vi "Get Dependencies.vi"(8 "error in (no error)":errorcluster, 11 "Device Ref in":T5 format="%.0x") -> (0 "error out":errorcluster, 2 "Dependencies":T1[](array[typedef]), 3 "Dev Ref out":T5 format="%.0x")   [LabVIEW 2011, in "TDMS Custom Device.lvlib"]
uses:
  TDMS Custom Device.lvlib
  <vilib>/NI Veristand/Custom Device API/Custom Device Item Ref.ctl
  <vilib>/NI Veristand/Custom Device API/Custom Device File Dependency.ctl
  <vilib>/NI Veristand/Custom Device API/Path Specification.ctl
  <vilib>/NI Veristand/Custom Device API/Path Type.ctl
  <vilib>/NI Veristand/Custom Device API/Custom Device Supported Target.ctl
  NationalInstruments.VeriStand.SystemStorage
  <vilib>/NI Veristand/Custom Device API/Custom Device API.lvlib
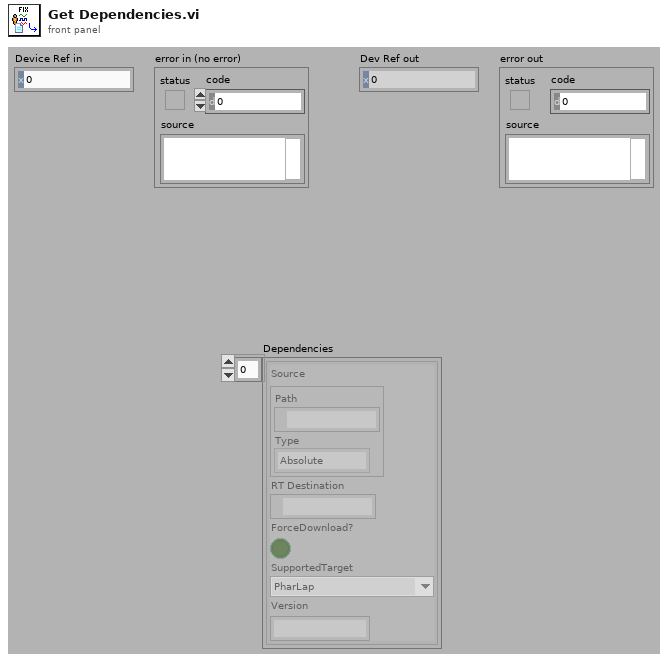
[diagram p1: front panel]
types:
  T1 = typedef "Custom Device API.lvlib/Custom Device File Dependency.ctl" = cluster{"Source":T2, "RT Destination":path, "ForceDownload?":bool, "SupportedTarget":T4, "Version":string}
  T2 = typedef "Custom Device API.lvlib/Path Specification.ctl" = cluster{"Path":path, "Type":T3}
  T3 = typedef "Custom Device API.lvlib/Path Type.ctl" = enum16{"Absolute", "To Base", "To Common Data Dir", "To Application Data Dir"}
  T4 = typedef "Custom Device API.lvlib/Custom Device Supported Target.ctl" = enum16{"All", "PharLap", "VxWorks", "Windows", "PharLap & Windows", "PharLap & VxWorks", "VxWorks & Windows"}
  T5 = typedef "Custom Device API.lvlib/Custom Device Item Ref.ctl" = u64
  T6 = typedef "Custom Device API.lvlib/Custom Device Pointer.ctl" = refnum<k24>
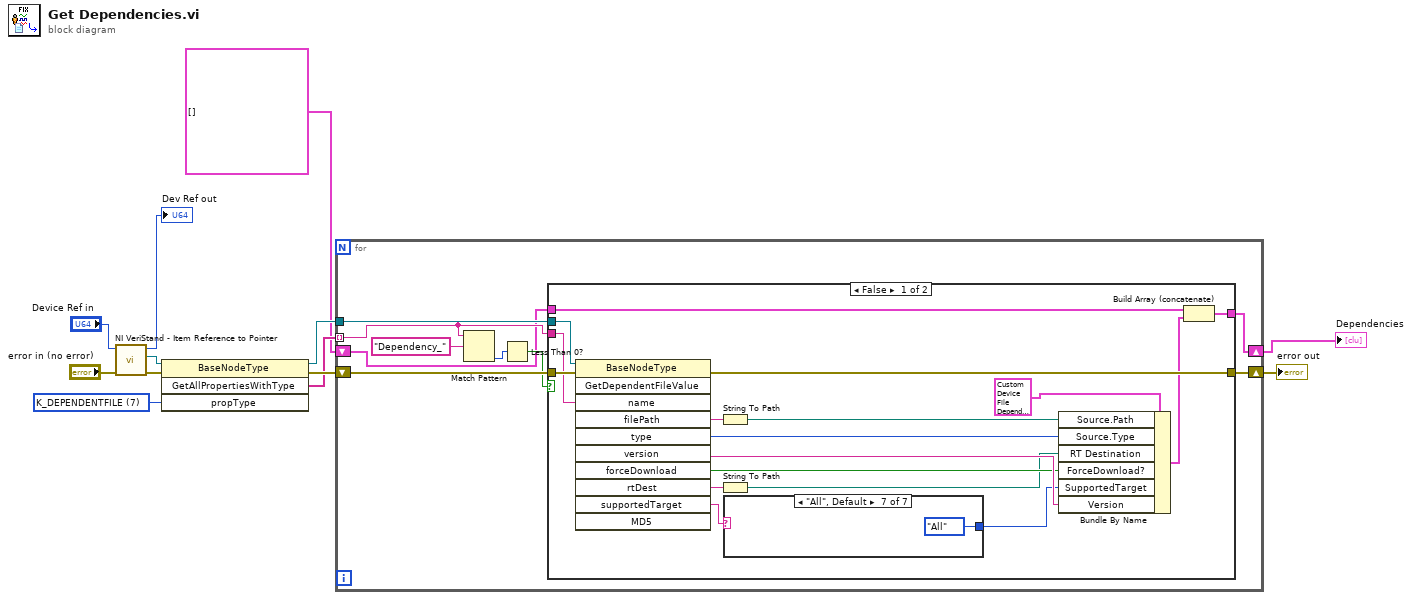
[diagram p0: block diagram]
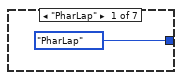
[diagram p2: hidden frame]
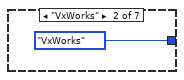
[diagram p3: hidden frame]
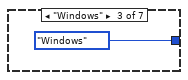
[diagram p4: hidden frame]
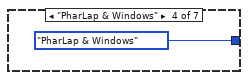
[diagram p5: hidden frame]
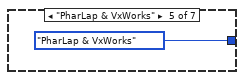
[diagram p6: hidden frame]
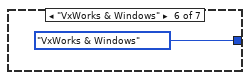
[diagram p7: hidden frame]
diagram:
  w7 = 7 items=["K_STRING", "K_BOOL", "K_I32", "K_U32", "K_DOUBLE", "K_U64", "K_VARIANT", "K_DEPENDENTFILE", "K_DEPENDENTNODE", "K_DATASOURCENODE", "K_U16", "K_DBLARR", "K_U32ARR", "K_I32ARR", "K_STRINGARR", "K_DICTIONARY", "K_DICTIONARYARR", "K_BINARYSTRING"] ("propType")
  n1 = call <vilib>:"NI VeriStand - Item Reference to Pointer.vi"("error in (no error)"="error in (no error)", "Item Ref in"="Device Ref in") -> ("error out"=w6:errorcluster, "Node Pointer"=w8:T6, "Item Ref out"=→"Dev Ref out":T5)  [unwired: 6 in, 1 out]
  n2 = invoke class="BaseNodeType" method="GetAllPropertiesWithType"(reference=w8, error in=w6, "propType"=w7) -> (reference out=w4:T6, error out=w5:errorcluster, "GetAllPropertiesWithType"=w3:string[])  [unwired: 1 in, 1 out]
  n3 = for {
    shift-right: [w20] -> w12
    shift-left: w5 -> [w21]
    tunnel: w4 -> [w19]
    tunnel: w3 -> [w15] mode=indexing
    shift-right: [w13] -> w1
    shift-left: T1[] [] ("Dependencies") -> [w14]
    n4 = Match Pattern(string=w15, regular expression="Dependency_") -> (offset past match=w17:i32)  [unwired: 1 in, 3 out]
    n5 = Less Than 0?(x=w17) -> (x < 0?=w16:bool)
    n6 = case shown="False" w16 {
      tunnel: w21 -> [w38 w47]
      tunnel: [w37 w47] -> w20
      tunnel: w19 -> [w36 _]
      tunnel: w15 -> [w35 _]
      tunnel: w14 -> [w33 w46]
      tunnel: [w31 w46] -> w13
      frame False {
        n7 = invoke class="BaseNodeType" method="GetDependentFileValue"(reference=w36, error in=w38, "name"=w35) -> (error out=w37:errorcluster, "filePath"=w30:string, "type"=w28:i32, "version"=w27:string, "forceDownload"=w26:bool, "rtDest"=w25:string, "supportedTarget"=w23:string)  [unwired: 8 in, 4 out]
        n8 = String To Path(string=w30) -> (path=w29:path)
        n9 = String To Path(string=w25) -> (path=w24:path)
        n10 = case shown="\"All\", Default" w23 {
          tunnel: [Custom_Device_Supported_Target."PharLap" ("SupportedTarget") Custom_Device_Supported_Target."VxWorks" ("SupportedTarget") Custom_Device_Supported_Target."Windows" ("SupportedTarget") Custom_Device_Supported_Target."PharLap & Windows" ("SupportedTarget") Custom_Device_Supported_Target."PharLap & VxWorks" ("SupportedTarget") Custom_Device_Supported_Target."VxWorks & Windows" ("SupportedTarget") Custom_Device_Supported_Target."All" ("SupportedTarget")] -> w22
          frame "PharLap" {
          }
          frame "VxWorks" {
          }
          frame "Windows" {
          }
          frame "PharLap & Windows" {
          }
          frame "PharLap & VxWorks" {
          }
          frame "VxWorks & Windows" {
          }
          frame "All", Default {
          }
        }
        n11 = Bundle By Name(cluster=T1 {"Source"={"Path"=path "", "Type"=enum."Absolute"}, "RT Destination"=path "", "ForceDownload?"=FALSE, "SupportedTarget"=enum."PharLap", "Version"=""} ("Dependency"), "Source.Path"=w29, "Source.Type"=w28, "RT Destination"=w24, "ForceDownload?"=w26, "SupportedTarget"=w22, "Version"=w27) -> (w32:T1)
        n12 = Build Array (concatenate)(w33, w32) -> (w31:T1[])
      }
      frame True {
      }
    }
  }
  "error out" <- w12
  "Dependencies" <- w1
